vi "OAT Verify Resampled Signal (OMP).vi"   [LabVIEW 2017, in "SoundVib_Resampling.lvlib"]
uses:
  <vilib>/addons/Sound and Vibration/Order Analysis/Resample Order Tracking/SoundVib_Resampling.lvlib
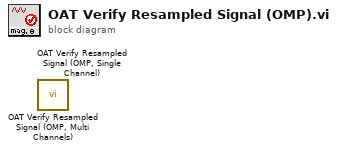
[diagram p0: block diagram]
diagram:
  n1 = call <vilib>:"OAT Verify Resampled Signal (OMP, Multi Channels).vi"() -> ()  [unwired: 10 in, 6 out]
  n2 = call <vilib>:"OAT Verify Resampled Signal (OMP, Single Channel).vi"() -> ()  [unwired: 10 in, 6 out]
